vi "TerminateErrorProcessor.vi"(7 "priority (-1, highest)":i32=-1, 8 "error in":errorcluster, 11 "error reporter in":refnum<class "ErrorReporter.lvclass">) -> (0 "error out":errorcluster, 2 "message sent?":bool)   [LabVIEW 2013, in "CLM_ErrorHandler.lvlib" / "ErrorReporter.lvclass"]
uses:
  ErrorReporter.lvclass
  ErrorReporter.lvclass/ErrorReporter.ctl
  <vilib>/CLM/LocalMessenger/PriorityLocalMessage/CLM_PriorityLocalMessage.lvclass/CLM_PriorityLocalMessage.ctl
  <vilib>/CLM/LocalMessenger/LocalMessage_Queue/CLM_LocalMessage_Queue.lvclass/CLM_LocalMessage_Queue.ctl
  <vilib>/CLM/LocalMessenger/PriorityLocalMessage/SendMessage.vi
  <vilib>/CLM/LocalMessenger/PriorityLocalMessage/SendMessageCluster.vi
  <vilib>/CLM/LocalMessenger/LocalMessage/BundleMessageCluster.vi
  <vilib>/CLM/LocalMessenger/LocalMessage_Queue/SendQueueMessage_Cluster.vi
  <vilib>/CLM/LocalMessenger/PriorityLocalMessage/BufferIndexToPriority.vi
  <vilib>/CLM/LocalMessenger/PriorityLocalMessage/PriorityToBufferIndex.vi
  <vilib>/CLM/LocalMessenger/PriorityLocalMessage/CLM_PriorityLocalMessage.lvclass
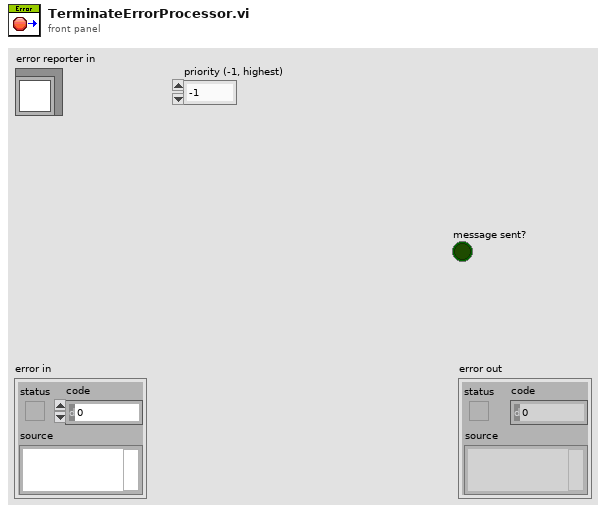
[diagram p1: front panel]
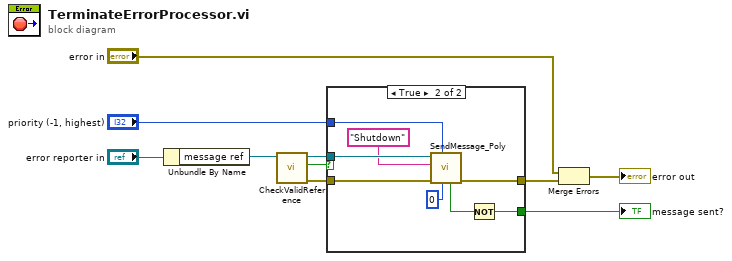
[diagram p0: block diagram]
diagram:
  n1 = Unbundle By Name("error reporter in") -> ("message ref"=w9:refnum<class "CLM_PriorityLocalMessage.lvclass">)
  n2 = call <vilib>:"CheckValidReference.vi"("message ref in"=w9) -> ("error out"=w6:errorcluster, "valid?"=w8:bool, "message ref out"=w7:refnum<class "CLM_PriorityLocalMessage.lvclass">)  [unwired: 8 in]
  n3 = case shown="True" w8 {
    tunnel: w7 -> [_ w19]
    tunnel: w6 -> [w11 w18]
    tunnel: "priority (-1, highest)" -> [_ w15]
    tunnel: [w11 w14] -> w4
    tunnel: [_ w12] -> w1
    frame False {
    }
    frame True {
      n4 = call-poly <vilib>:"SendMessage_Poly.vi"("timeout in ms (-1)"=0, "priority (-1, highest)"=w15, "error in"=w18, "name"="Shutdown", "message ref in"=w19) -> ("error out"=w14:errorcluster, "timed out?"=w13:bool)  [unwired: 3 in, 2 out]
      n5 = Not(x=w13) -> (.not. x?=w12:bool)
    }
  }
  "message sent?" <- w1
  n6 = Merge Errors("error in", w4) -> (→"error out":errorcluster)
